vi "_Test, Set Table Size.vi"() -> ()   [LabVIEW 2024, in "EQMF.lvlib" / "Controls.lvlib"]
uses:
  Controls.lvlib
panel:
  in  "Aspect Ratio":cluster{"W/H":dbl, "Enable":bool}={"W/H"=1.0, "Enable"=FALSE} {"W/H" format="%.2g"}
  in  "Min Size":cluster{"Width":i32, "Height":i32}={"Width"=250, "Height"=200}
  out "error out":errorcluster
  in  "dY":i32=40
  in  "dX":i32=40
  in  "Tab Control":enum32{"Page 1", "Page 2"}(tab)
  out "TableX":string[][](table) caption="GPS Satellites"
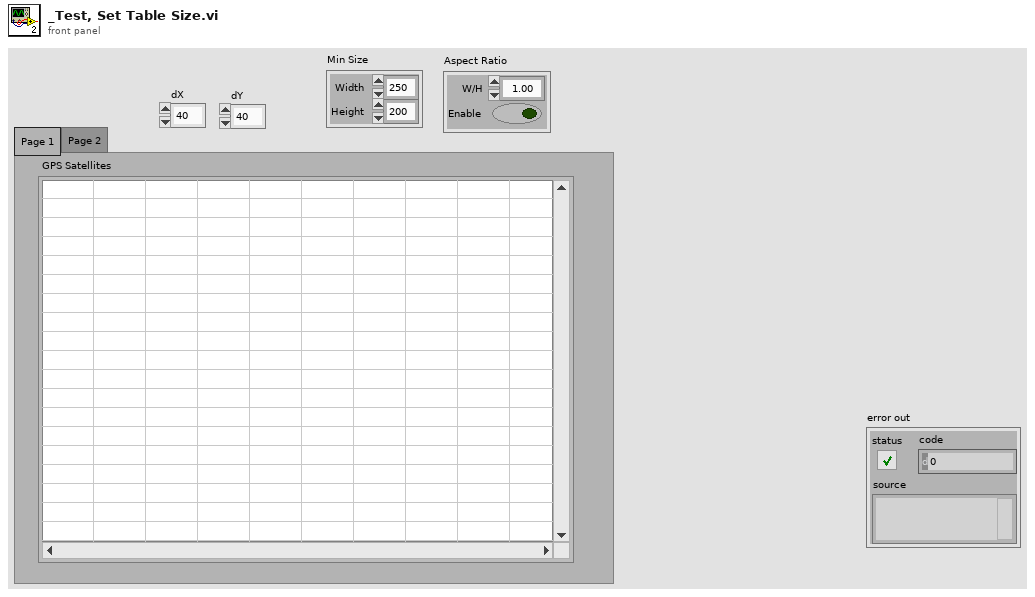
[diagram p1: front panel]
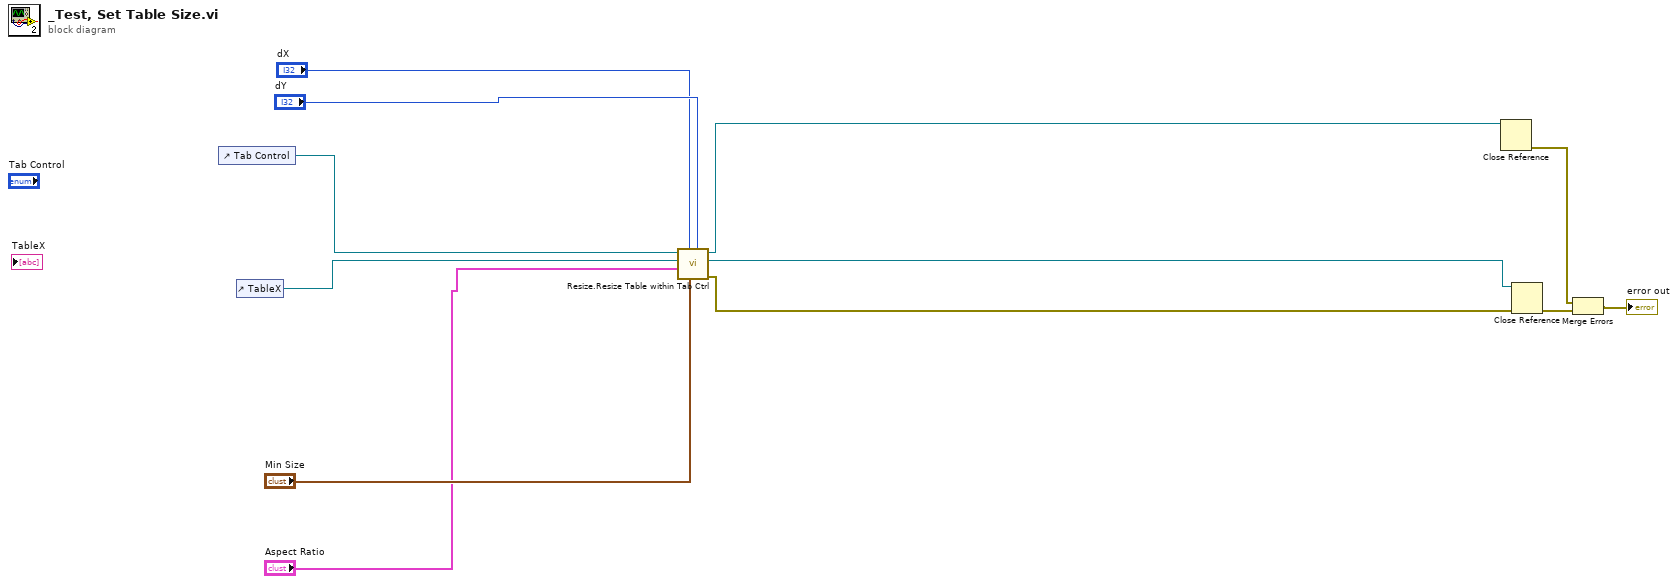
[diagram p0: block diagram]
diagram:
  n1 = control-ref of="Tab Control"() -> (w9:refnum<vi>)
  n2 = control-ref of="TableX"() -> (w8:refnum<vi>)
  n3 = call "Resize.Resize Table within Tab Ctrl.vi"("Pix from Bottom"="dY", "Min Size"="Min Size", "Pix from Right"="dX", "Aspect Ratio"="Aspect Ratio", "Table Ctrl"=w8, "Tab Ctrl"=w9) -> ("error out"=w3:errorcluster, "Table Ctrl Out"=w5:refnum<vi>, "Tab Ctrl Out"=w4:refnum<vi>)  [unwired: 3 in]
  n4 = Close Reference(reference=w4) -> (error out=w11:errorcluster)  [unwired: 1 in]
  n5 = Close Reference(reference=w5, error in (no error)=w3) -> (error out=w12:errorcluster)
  n6 = Merge Errors(w11, w12) -> (→"error out":errorcluster)
